vi "Search or Split String__ogtk.vi"(3 "offset (0)":i32, 4 "search string/char (-)":string, 5 "string":string) -> (0 "offset after match":i32, 1 "substring after match":string, 2 "substring before match":string)   [LabVIEW 2011]
doc: "Performs the standard Search/Split String function, but, in Search mode, splits string after search string/char and returns the offset after the match."
panel:
  # "[OpenG VI Tags] ***Do Not Remove***"
  # "Multicharacter Search or Split String.vi\n\nPerforms the standard Search/Split String function, but, in Search mode, splits string after search string/char and returns the offset after the match.\n\nPlease visit http://www.OpenG.org to learn about the\nOpen Source LabVIEW software movement.\n\nNOTICE -- YOU MUST LEAVE THIS NOTICE IN PLACE.  PER THE TERMS OF THE LICENSE BELOW, YOU MAY SUBLICENSE THIS SOFTWARE \nIN ANY WAY THAT DOES NOT CONFLICT WITH THIS LICENSE.\n\n### BSD License (http://www.opensource.org/licenses/bsd-license.php) Begin ###\n \nCopyright (c) 2005, MKS Instruments, Inc., author: Doug Femec<doug_femec@mksinst.com>, IM dafemec\n\nAll rights reserved.\n\nRedistribution and use in source and binary forms, with or without modification, are permitted provided that the following conditions are met:\n\n    * Redistributions of source code must retain the above copyright notice, this list of conditions and the following disclaimer.\n    * Redistributions in binary form must reproduce the above copyright notice, this list of conditions and the following disclaimer in the \n       documentation and/or other materials provided with the distribution.\n    * Neither the name of SciWare, James Kring, Inc., nor the names of its contributors may be used to endorse or promote products derived \n       from this software without specific prior written permission.\n\nTHIS SOFTWARE IS PROVIDED BY THE COPYRIGHT HOLDERS AND CONTRIBUTORS \"AS IS\" AND ANY EXPRESS OR IMPLIED WARRANTIES, \nINCLUDING, BUT NOT LIMITED TO, THE IMPLIED WARRANTIES OF MERCHANTABILITY AND FITNESS FOR A PARTICULAR PURPOSE ARE \nDISCLAIMED. IN NO EVENT SHALL THE COPYRIGHT OWNER OR CONTRIBUTORS BE LIABLE FOR ANY DIRECT, INDIRECT, INCIDENTAL,\n SPECIAL, EXEMPLARY, OR CONSEQUENTIAL DAMAGES (INCLUDING, BUT NOT LIMITED TO, PROCUREMENT OF SUBSTITUTE GOODS OR \nSERVICES; LOSS OF USE, DATA, OR PROFITS; OR BUSINESS INTERRUPTION) HOWEVER CAUSED AND ON ANY THEORY OF LIABILITY, \nWHETHER IN CONTRACT, STRICT LIABILITY, OR TORT (INCLUDING NEGLIGENCE OR OTHERWISE) ARISING IN ANY WAY OUT OF THE USE \nOF THIS SOFTWARE, EVEN IF ADVISED OF THE POSSIBILITY OF SUCH DAMAGE.\n\n### BSD License End ###"
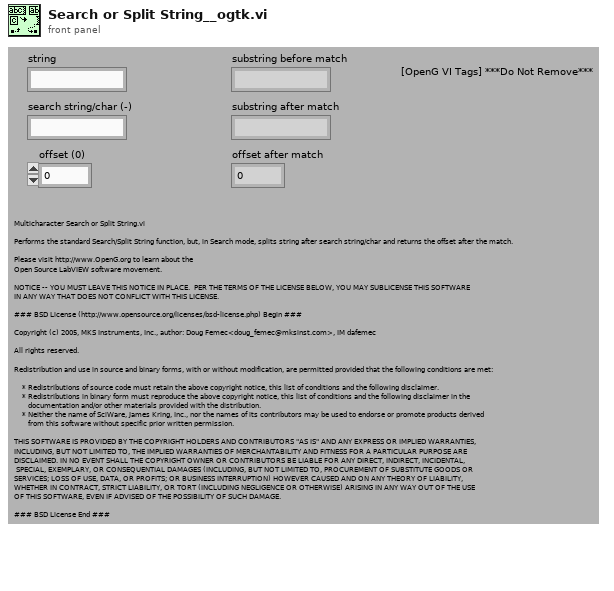
[diagram p1: front panel]
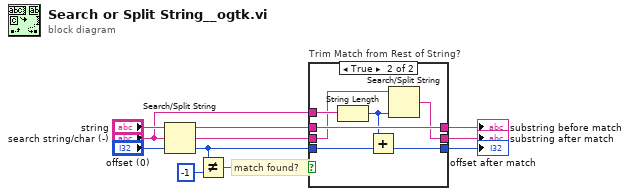
[diagram p0: block diagram]
diagram:
  # "match found?"
  n1 = Search/Split String(string="string", search string/char (-)="search string/char (-)", offset (0)="offset (0)") -> (substring before match=w8:string, match + rest of string=w7:string, offset of match=w1:i32)
  n2 = Not Equal?(x=w1, y=-1) -> (x != y?=w2:bool)
  n3 = case "Trim Match from Rest of String?" shown="True" w2 {
    tunnel: "search string/char (-)" -> [_ w21]
    tunnel: w8 -> [w14 w20]
    tunnel: w7 -> [w13 w19]
    tunnel: [w12 w17] -> w6
    tunnel: [w14 w20] -> w5
    tunnel: [w13 w16] -> w4
    tunnel: w1 -> [w12 w15]
    frame False {
    }
    frame True {
      n4 = String Length(string=w21) -> (length=w18:i32)
      n5 = Add(x=w18, y=w15) -> (x+y=w17:i32)
      n6 = Search/Split String(string=w19, offset (0)=w18) -> (match + rest of string=w16:string)  [unwired: 1 in, 2 out]
    }
  }
  "offset after match" <- w6
  "substring after match" <- w4
  "substring before match" <- w5
